vi "Update Pin Map from XML.vi"(8 "error in":errorcluster, 11 "request data":T2) -> (0 "error out":errorcluster, 3 "response data":T1)   [LabVIEW 2021, in "NI Pin Map V1 Client.lvlib"]
uses:
  NI Pin Map V1 Client.lvlib
  gRPC/Generated APIs/ni/measurementlink/pinmap/v1/RPC Messages/ni_measurementlink_pinmap_v1_UpdatePinMapFromXmlRequest.ctl
  gRPC/Generated APIs/ni/measurementlink/pinmap/v1/RPC Messages/ni_measurementlink_pinmap_v1_PinMap.ctl
  Discovery V1/TypeDefs/gRPC Client Cache FGV Action.ctl
  gRPC/Generated APIs/ni/measurementlink/pinmap/v1/ni.measurementlink.pinmap.v1.api.lvlib
  Discovery V1/NI Discovery V1 Client.lvlib
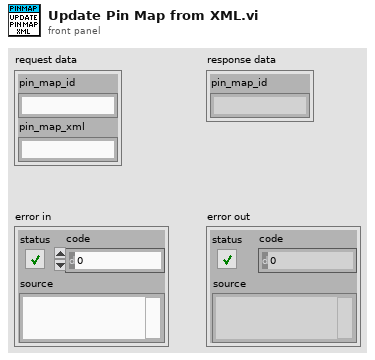
[diagram p1: front panel]
types:
  T1 = typedef "ni.measurementlink.pinmap.v1.api.lvlib/ni_measurementlink_pinmap_v1_PinMap.ctl" = cluster{"pin_map_id":string}
  T2 = typedef "ni.measurementlink.pinmap.v1.api.lvlib/ni_measurementlink_pinmap_v1_UpdatePinMapFromXmlRequest.ctl" = cluster{"pin_map_id":string, "pin_map_xml":string}
  T3 = typedef "NI Discovery V1 Client.lvlib/gRPC Client Cache FGV Action.ctl" = enum16{"Get Client", "Recreate Client", "Destroy Client", "Update ClusterId"}
  T4 = typedef "grpc-lvsupport-release.lvlib/grpcId.ctl" = u64
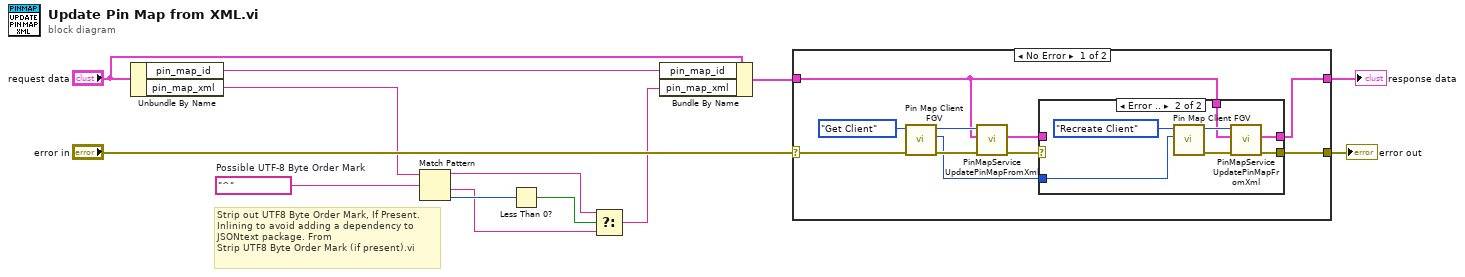
[diagram p0: block diagram]
diagram:
  w1 = "^﻿"  # Possible UTF-8 Byte Order Mark
  # "Strip out UTF8 Byte Order Mark, If Present.\nInlining to avoid adding a dependency to\nJSONtext package. From\nStrip UTF8 Byte Order Mark (if present).vi"
  n1 = Unbundle By Name("request data") -> ("pin_map_id"=w9:string, "pin_map_xml"=w8:string)
  n2 = Match Pattern(string=w8, regular expression=w1) -> (before substring=w4:string, after substring=w2:string, offset past match=w5:i32)  [unwired: 1 in, 1 out]
  n3 = Less Than 0?(x=w5) -> (x < 0?=w3:bool)
  n4 = Select(t=w4, s=w3, f=w2) -> (s? t:f=w7:string)
  n5 = Bundle By Name(cluster="request data", "pin_map_id"=w9, "pin_map_xml"=w7) -> (w6:T2)
  n6 = case shown="No Error" "error in" {
    selector: "error in" -> [w23 w33]
    tunnel: [w19 w33] -> w12
    tunnel: w6 -> [w14 _]
    tunnel: [w17 _] -> w11
    frame No Error {
      n7 = call "Pin Map Client FGV.vi"("error in"=w23, "action"=gRPC_Client_Cache_FGV_Action."Get Client") -> ("error out"=w22:errorcluster, "unique id out"=w15:u64, "grpc client id"=w21:T4)  [unwired: 7 in]
      n8 = call "PinMapService UpdatePinMapFromXml.vi"("error in"=w22, "Request Data"=w14, "gRPC ID"=w21) -> ("error out"=w20:errorcluster, "Response Data"=w16:T1)  [unwired: 6 in, 1 out]
      n9 = case shown="Error .." w20 {
        selector: w20 -> [w25 _]
        tunnel: [w25 w29] -> w19
        tunnel: [w24 w28] -> w17
        tunnel: w16 -> [w24 _]
        tunnel: w15 -> [_ w27]
        tunnel: w14 -> [_ w26]
        frame No Error {
        }
        frame Error {
          n10 = call "Pin Map Client FGV.vi"("unique id in"=w27, "action"=gRPC_Client_Cache_FGV_Action."Recreate Client") -> ("error out"=w30:errorcluster, "grpc client id"=w31:T4)  [unwired: 7 in, 1 out]
          n11 = call "PinMapService UpdatePinMapFromXml.vi"("error in"=w30, "Request Data"=w26, "gRPC ID"=w31) -> ("error out"=w29:errorcluster, "Response Data"=w28:T1)  [unwired: 6 in, 1 out]
        }
      }
    }
    frame Error {
    }
  }
  "error out" <- w12
  "response data" <- w11
